vi "Configure Acquisition.vi"(5 "sweep mode continuous (Off)":bool, 6 "number of sweeps":i32 format="%.0g", 7 "detector type (Auto Peak)":i32(ring)=1 items=["Auto Peak"=1, "Average"=2, "Maximum Peak"=3, "Minimum Peak"=4, "Sample"=5, "RMS"=6], 8 "error in (no error)":errorcluster {"code" format="%.0x"}, 9 "vertical scale (Linear)":i32(ring)=1 items=["Linear"=1, "Logarithmic"=2], 10 "detector type auto (Off)":bool, 11 "instrument handle":refnum<k15>) -> (0 "error out":errorcluster {"code" format="%.0x"}, 3 "instrument handle out":refnum<k15>)   [LabVIEW 2009, in "Keysight XSAn.lvlib"]
doc: "This function configures the acquisition attributes of the IviSpecAn.\n\nSupported Models: M9290A, N8973B, N8974B, N8975B, N8976B, N9000A, N9000B, N9010A, N9010B, N9020A, N9020B, N9030A, N9030B, N9038A, N9040B, N9041B, SPN9003A, SPN9026A"
uses:
  <instrlib>/Keysight XSAn/Keysight XSAn.lvlib
  AgXSAn.dll
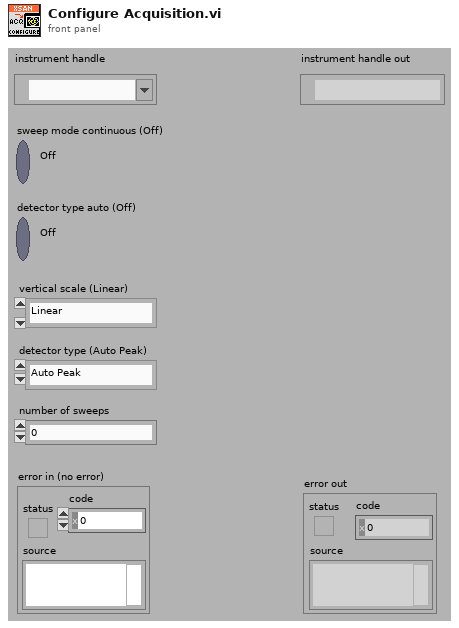
[diagram p1: front panel]
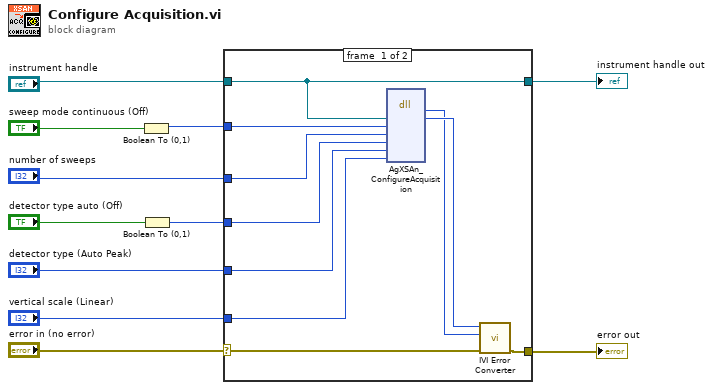
[diagram p0: block diagram]
diagram:
  n1 = Boolean To (0,1)(Boolean="sweep mode continuous (Off)") -> (0, 1=w5:i16)
  n2 = Boolean To (0,1)(Boolean="detector type auto (Off)") -> (0, 1=w3:i16)
  n3 = case shown="No Error" "error in (no error)" {
    selector: "error in (no error)" -> [w19 w23]
    tunnel: [w20 w23] -> w10
    tunnel: "instrument handle" -> [w17 w22]
    tunnel: [w17 w22] -> w8
    tunnel: w5 -> [w16 _]
    tunnel: "number of sweeps" -> [w15 _]
    tunnel: w3 -> [w14 _]
    tunnel: "detector type (Auto Peak)" -> [w13 _]
    tunnel: "vertical scale (Linear)" -> [w12 _]
    frame #0 {
      n4 = dll-call lib="AgXSAn**.dll" fn="AgXSAn_ConfigureAcquisition" ("LabVIEW:IviSpecAn_ConfigureAcquisition")("instrument handle"=w17, "sweep mode continuous"=w16, "number of sweeps"=w15, "detector type auto"=w14, "detector type"=w13, "vertical scale"=w12) -> ("Status"=w18:i32, "instrument handle"=w21:u32)  [unwired: 8 in, 2 out]
      n5 = call <instrlib>:"IVI Error Converter.vi"("error in (no error)"=w19, "IVI error code (0)"=w18, "instrument handle"=w21) -> ("error out"=w20:errorcluster)  [unwired: 7 in, 1 out]
    }
    frame #1 {
    }
  }
  "error out" <- w10
  "instrument handle out" <- w8
